vi "Excel Report.vi"(0 "标题配置":cluster{"title":string, "font":T2}={"title"="测试报告", "font"={"font name"="", "font size"=24.0, "bold"=2, "italic"=2, "underline"=2, "strike through"=2, "font color"=16777222}} {"font"."font size" format="%0.2f"; "font"."strike through" items=["Unchanged", "Yes", "No"]; "font"."underline" items=["Unchanged", "Yes", "No"]; "font"."italic" items=["Unchanged", "Yes", "No"]; "font"."bold" items=["Unchanged", "Yes", "No"]}, 1 "测试信息":cluster{"font":T2, "字符串":string}={"font"={"font name"="", "font size"=12.0, "bold"=2, "italic"=2, "underline"=2, "strike through"=2, "font color"=16777222}, "字符串"=""} {"font"."font size" format="%0.2f"; "font"."strike through" items=["Strk Unchanged", "Strk Yes", "Strk No"]; "font"."underline" items=["Und Unchanged", "Und Yes", "Und No"]; "font"."italic" items=["Ital Unchanged", "Ital Yes", "Ital No"]; "font"."bold" items=["Bold Unchanged", "Bold Yes", "Bold No"]}, 2 "文本":cluster{"font":T2, "字符串":string}={"font"={"font name"="", "font size"=12.0, "bold"=2, "italic"=2, "underline"=2, "strike through"=2, "font color"=16777222}, "字符串"=""} {"font"."font size" format="%0.2f"; "font"."strike through" items=["Strk Unchanged", "Strk Yes", "Strk No"]; "font"."underline" items=["Und Unchanged", "Und Yes", "Und No"]; "font"."italic" items=["Ital Unchanged", "Ital Yes", "Ital No"]; "font"."bold" items=["Bold Unchanged", "Bold Yes", "Bold No"]}, 3 "表格":T3={"auto format"=11, "font"={"font name"="", "font size"=0.0, "bold"=0, "italic"=0, "underline"=0, "strike through"=0, "font color"=0}, "表格 2"=[["1", "1.5", "5.6", "5.6", "7.9", "4.6"], ["2", "2.5", "7.6", "6.5", "7.2", "7.5"], ["3", "6.8", "9.1", "4.2", "6.2", "6.1"], ["4", "6.7", "7.1", "7.2", "1.0", "8.3"], ["5", "6.4", "4.3", "9.2", "5.8", "4.2"], ["6", "8.6", "8.2", "4.3", "8.6", "4.5"]]} {"auto format" items=["xlRangeAutoFormat3DEffects1"=13, "xlRangeAutoFormat3DEffects2"=14, "xlRangeAutoFormatAccounting1"=4, "xlRangeAutoFormatAccounting2"=5, "xlRangeAutoFormatAccounting3"=6, "xlRangeAutoFormatAccounting4"=17, "xlRangeAutoFormatClassic1"=1, "xlRangeAutoFormatClassic2"=2, "xlRangeAutoFormatClassic3"=3, "xlRangeAutoFormatColor1"=7, "xlRangeAutoFormatColor2"=8, "xlRangeAutoFormatColor3"=9, "xlRangeAutoFormatList1"=10, "xlRangeAutoFormatList2"=11, "xlRangeAutoFormatList3"=12, "xlRangeAutoFormatLocalFormat1"=15, "xlRangeAutoFormatLocalFormat2"=16, "xlRangeAutoFormatLocalFormat3"=19, "xlRangeAutoFormatLocalFormat4"=20, "xlRangeAutoFormatReport1"=21, "xlRangeAutoFormatReport2"=22, "xlRangeAutoFormatReport3"=23, "xlRangeAutoFormatReport4"=24, "xlRangeAutoFormatReport5"=25, "xlRangeAutoFormatReport6"=26, "xlRangeAutoFormatReport7"=27, "xlRangeAutoFormatReport8"=28, "xlRangeAutoFormatReport9"=29, "xlRangeAutoFormatReport10"=30, "xlRangeAutoFormatClassicPivotTable"=31, "xlRangeAutoFormatTable1"=32, "xlRangeAutoFormatTable2"=33, "xlRangeAutoFormatTable3"=34, "xlRangeAutoFormatTable4"=35, "xlRangeAutoFormatTable5"=36, "xlRangeAutoFormatTable6"=37, "xlRangeAutoFormatTable7"=38, "xlRangeAutoFormatTable8"=39, "xlRangeAutoFormatTable9"=40, "xlRangeAutoFormatTable10"=41, "xlRangeAutoFormatPTNone"=42, "xlRangeAutoFormatNone"=-4142, "xlRangeAutoFormatSimple"=-4154]; "font"."font size" format="%0.2f"; "font"."strike through" items=["Strk Unchanged", "Strk Yes", "Strk No"]; "font"."underline" items=["Und Unchanged", "Und Yes", "Und No"]; "font"."italic" items=["Ital Unchanged", "Ital Yes", "Ital No"]; "font"."bold" items=["Bold Unchanged", "Bold Yes", "Bold No"]}, 4 "图表配置":T4={"chart type"=4, "graph title (\"\")"="测试图表"} {"chart type" items=["xlColumnClustered"=51, "xlColumnStacked"=52, "xlColumnStacked100"=53, "xl3DColumnClustered"=54, "xl3DColumnStacked"=55, "xl3DColumnStacked100"=56, "xlBarClustered"=57, "xlBarStacked"=58, "xlBarStacked100"=59, "xl3DBarClustered"=60, "xl3DBarStacked"=61, "xl3DBarStacked100"=62, "xlLineStacked"=63, "xlLineStacked100"=64, "xlLineMarkers"=65, "xlLineMarkersStacked"=66, "xlLineMarkersStacked100"=67, "xlPieOfPie"=68, "xlPieExploded"=69, "xl3DPieExploded"=70, "xlBarOfPie"=71, "xlXYScatterSmooth"=72, "xlXYScatterSmoothNoMarkers"=73, "xlXYScatterLines"=74, "xlXYScatterLinesNoMarkers"=75, "xlAreaStacked"=76, "xlAreaStacked100"=77, "xl3DAreaStacked"=78, "xl3DAreaStacked100"=79, "xlDoughnutExploded"=80, "xlRadarMarkers"=81, "xlRadarFilled"=82, "xlSurface"=83, "xlSurfaceWireframe"=84, "xlSurfaceTopView"=85, "xlSurfaceTopViewWireframe"=86, "xlBubble"=15, "xlBubble3DEffect"=87, "xlStockHLC"=88, "xlStockOHLC"=89, "xlStockVHLC"=90, "xlStockVOHLC"=91, "xlCylinderColClustered"=92, "xlCylinderColStacked"=93, "xlCylinderColStacked100"=94, "xlCylinderBarClustered"=95, "xlCylinderBarStacked"=96, "xlCylinderBarStacked100"=97, "xlCylinderCol"=98, "xlConeColClustered"=99, "xlConeColStacked"=100, "xlConeColStacked100"=101, "xlConeBarClustered"=102, "xlConeBarStacked"=103, "xlConeBarStacked100"=104, "xlConeCol"=105, "xlPyramidColClustered"=106, "xlPyramidColStacked"=107, "xlPyramidColStacked100"=108, "xlPyramidBarClustered"=109, "xlPyramidBarStacked"=110, "xlPyramidBarStacked100"=111, "xlPyramidCol"=112, "xl3DColumn"=-4100, "xlLine"=4, "xl3DLine"=-4101, "xl3DPie"=-4102, "xlPie"=5, "xlXYScatter"=-4169, "xl3DArea"=-4098, "xlArea"=1, "xlDoughnut"=-4120, "xlRadar"=-4151]}, 6 "报告类型":u16(ring)=2, 7 "簇":T1={"Save Report 2"=FALSE, "路径"=path "/Report.html", "Print Report 2"=FALSE, "份数"=1} {"份数" min=1 max=10 step=1}) -> ()   [LabVIEW 2015]
uses:
  <vilib>/addons/_office/_wordsub.llb/font.ctl
  <vilib>/addons/_office/excel.llb/Excel Easy Table (str).vi
  <vilib>/Utility/NIReport.llb/NI_report.lvclass
  <vilib>/addons/_office/NI_ReportGenerationToolkit.lvlib
  <vilib>/Utility/NIReport.llb/Excel/NI_Excel.lvclass
panel:
  out "表格 2":string[][](table)=[["1", "1.5", "5.6", "5.6", "7.9", "4.6"], ["2", "2.5", "7.6", "6.5", "7.2", "7.5"], ["3", "6.8", "9.1", "4.2", "6.2", "6.1"], ["4", "6.7", "7.1", "7.2", "1.0", "8.3"], ["5", "6.4", "4.3", "9.2", "5.8", "4.2"], ["6", "8.6", "8.2", "4.3", "8.6", "4.5"]]
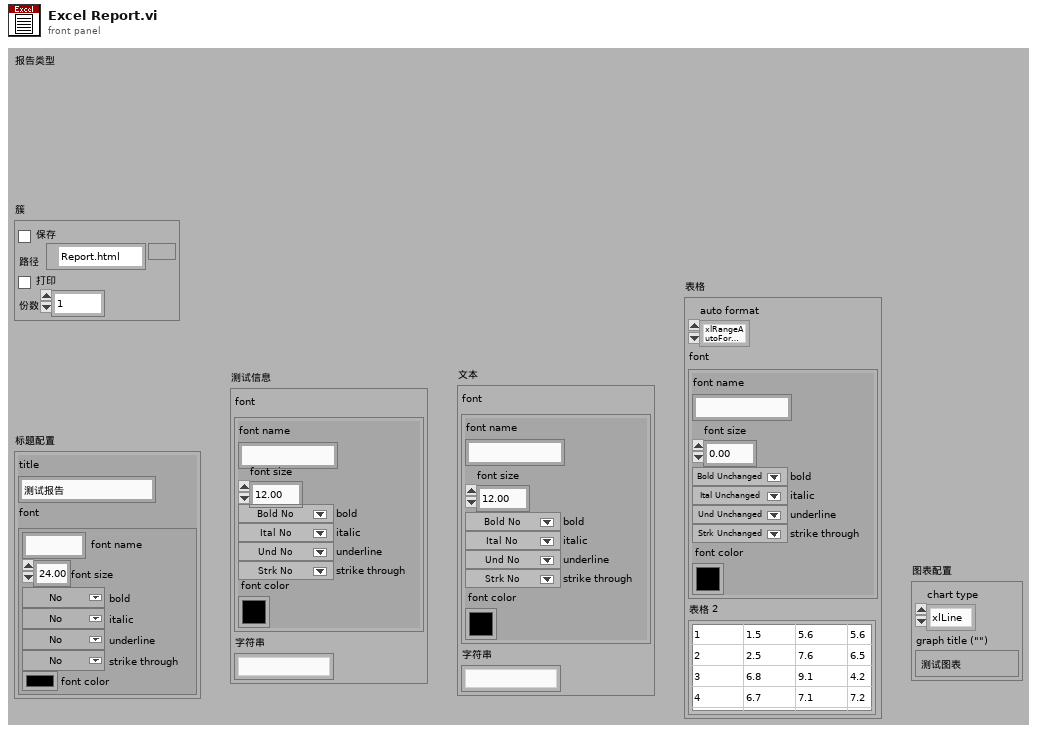
[diagram p1: front panel]
types:
  T1 = cluster{"Save Report 2":bool, "路径":path, "Print Report 2":bool, "份数":i32}
  T2 = typedef "font.ctl" = cluster{"font name":string, "font size":dbl, "bold":u16, "italic":u16, "underline":u16, "strike through":u16, "font color":u32}
  T3 = cluster{"auto format":i32, "font":T2, "表格 2":string[][]}
  T4 = cluster{"chart type":i32, "graph title (\"\")":string}
  T5 = typedef "Generate Report Object Reference.ctl" = refnum<class "NI_report.lvclass">
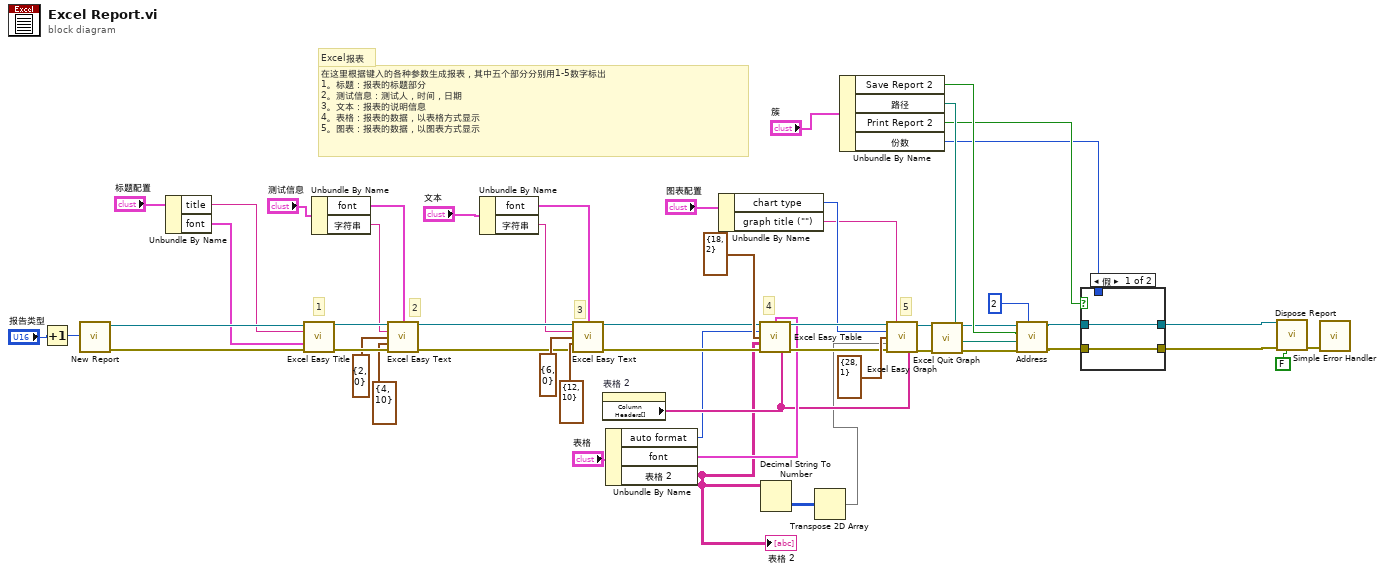
[diagram p0: block diagram]
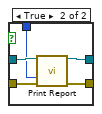
[diagram p2: hidden frame]
diagram:
  # "在这里根据键入的各种参数生成报表，其中五个部分分别用1-5数字标出\n1。标题：报表的标题部分\n2。测试信息：测试人，时间，日期\n3。文本：报表的说明信息\n4。表格：报表的数据，以表格方式显示\n5。图表：报表的数据，以图表方式显示"
  # "3"
  # "2"
  # "5"
  # "4"
  # "1"
  # "Excel报表"
  n1 = Increment(x="报告类型") -> (x+1=w23:u16)
  n2 = call <vilib>:"New Report.vi"("report type"=w23) -> ("report out"=w21:refnum<class "NI_report.lvclass">, "error out"=w20:errorcluster)  [unwired: 13 in]
  n3 = Unbundle By Name("标题配置") -> ("title"=w6:string, "font"=w12:T2)
  n4 = call <vilib>:"Excel Easy Title.vi"("report in"=w21, "title"=w6, "font"=w12, "error in (no error)"=w20) -> ("report out"=w49:refnum<class "NI_report.lvclass">, "error out"=w48:errorcluster)  [unwired: 9 in, 1 out]
  n5 = Unbundle By Name("测试信息") -> ("font"=w36:T2, "字符串"=w37:string)
  n6 = call <vilib>:"Excel Easy Text.vi"("report in"=w49, "font"=w36, "text"=w37, "start (-1, -1)"=cluster{"row":i32, "column":i32} {"row"=2, "column"=0} ("start"), "end (-1, -1)"=cluster{"row":i32, "column":i32} {"row"=4, "column"=10} ("end"), "error in (no error)"=w48) -> ("report out"=w43:refnum<class "NI_report.lvclass">, "error out"=w42:errorcluster)  [unwired: 5 in, 3 out]
  n7 = Unbundle By Name("文本") -> ("font"=w34:T2, "字符串"=w33:string)
  n8 = call <vilib>:"Excel Easy Text.vi"("report in"=w43, "font"=w34, "text"=w33, "start (-1, -1)"=cluster{"row":i32, "column":i32} {"row"=6, "column"=0} ("start"), "end (-1, -1)"=cluster{"row":i32, "column":i32} {"row"=12, "column"=10} ("end"), "error in (no error)"=w42) -> ("report out"=w41:refnum<class "NI_report.lvclass">, "error out"=w40:errorcluster)  [unwired: 5 in, 3 out]
  n9 = property on="表格 2" class="Tbl (严格)"() -> ("Column Headers[]"=w26:string[])  [unwired: 2 in, 2 out]
  n10 = Unbundle By Name("表格") -> ("auto format"=w1:i32, "font"=w30:T2, "表格 2"=w24:string[][])
  "表格 2" <- w24
  n11 = Unbundle By Name("图表配置") -> ("chart type"=w29:i32, "graph title (\"\")"=w28:string)
  n12 = call-poly <vilib>:"Excel Easy Table.vi"("report in"=w41, "font"=w30, "auto format (none)"=w1, "start (0, 0)"=cluster{"row":i32, "column":i32} {"row"=18, "column"=2} ("position"), "text data"=w24, "error in (no error)"=w40, "column headers"=w26) -> ("report out"=w51:refnum<class "NI_report.lvclass">, "error out"=w50:errorcluster)  [unwired: 4 in, 3 out]
  n13 = Decimal String To Number(string=w24) -> (number=w27:i32[][])  [unwired: 2 in, 1 out]
  n14 = Transpose 2D Array(2D array=w27) -> (transposed array=w25:i32[][])
  n15 = Unbundle By Name("簇") -> ("Save Report 2"=w10:bool, "路径"=w9:path, "Print Report 2"=w8:bool, "份数"=w7:i32)
  n16 = call <vilib>:"Excel Easy Graph.vi"("report in"=w51, "graph title (\"\")"=w28, "graph type (col clustered)"=w29, "start (0, 0)"=cluster{"row":i32, "column":i32} {"row"=28, "column"=1} ("position"), "data"=w25, "error in (no error)"=w50, "column headers"=w26) -> ("report out"=w5:refnum<class "NI_report.lvclass">, "error out"=w3:errorcluster)  [unwired: 7 in]
  n17 = call <vilib>:"Excel Quit Graph.vi"("report in"=w5, "error in (no error)"=w3) -> ("report out"=w4:refnum<class "NI_report.lvclass">, "error out"=w2:errorcluster)  [unwired: 12 in]
  n18 = call "Address.vi"("报告类型"=u16 2, "错误簇输入"=w2, "路径"=w9, "保存？"=w10, "报告输入"=w4) -> ("错误簇输出"=w18:errorcluster, "报告输出"=w17:T5)  [unwired: 5 in]
  n19 = case shown="假" w8 {
    tunnel: w18 -> [w54 w58]
    tunnel: w17 -> [w55 w57]
    tunnel: [w55 w59] -> w15
    tunnel: [w54 w60] -> w13
    tunnel: w7 -> [_ w56]
    frame False {
    }
    frame True {
      n20 = call-dynamic "Print Report.vi"("report in"=w57, "number of copies (1)"=w56, "error in (no error)"=w58) -> ("report out"=w59:T5, "error out"=w60:errorcluster)  [unwired: 11 in]
    }
  }
  n21 = call-dynamic "Dispose Report.vi"("report in"=w15, "error in (no error)"=w13, "close report? (T)"=FALSE ("Close Report? (T)")) -> ("error out"=w14:errorcluster)  [unwired: 12 in]
  n22 = call <vilib>:"Simple Error Handler.vi"("error in (no error)"=w14) -> ()  [unwired: 4 in, 5 out]
